vi "Set Busy Cursor.vi"() -> ()   [LabVIEW 2023]
doc: "This VI demonstrates how to set the cursor to the busy cursor. Clicking the Set Busy button will change the cursor to the busy cursor. You will still be able to click on other buttons on the user interface. Clicking the Set Busy and Disable button will set the cursor to busy and disable the cursor. During this time, all user interface events will be ignored. After 5 seconds, Unset Busy.vi will be called and the cursor will no longer be busy.\n\nThe default and busy cursors are going to be OS dependent. If a cursor that does not depend on OS is needed, Set Cursor.vi should be used instead of Set/Unset Busy. In this case, you will not be able to disable clicking.\n\nIn a real application, if the cursor is set to disable clicking, there should be some way to ensure that Unset Busy.vi can be called. Otherwise, the only way to stop the VI is to use the Abort Execution button. \n\nThis example shows a usage of the Simple State Machine project template."
uses:
  controls/Set Busy Cursor State.ctl
panel:
  out "Busy Progress":u32(slide) scale=0.0..5000.0
  in  "Button":bool
  in  "Set Busy and Disable":bool
  in  "Stop":bool
  in  "Set Busy":bool
  # "Overview: Demonstrates the use of the Cursor VIs to set a busy cursor.\nInstructions:\n1. Run the VI.\n2. Click the Set Busy button. While the Busy Progress bar is incrementing, click the Button. Notice that its value changes.\n3. After the Busy Progress is complete, click the Set Busy and Disable button. While the Busy Progress bar is incrementing, click the Button. Since busy cursor clicks are disabled, the value will not change.\n4. Click Stop to stop the VI."
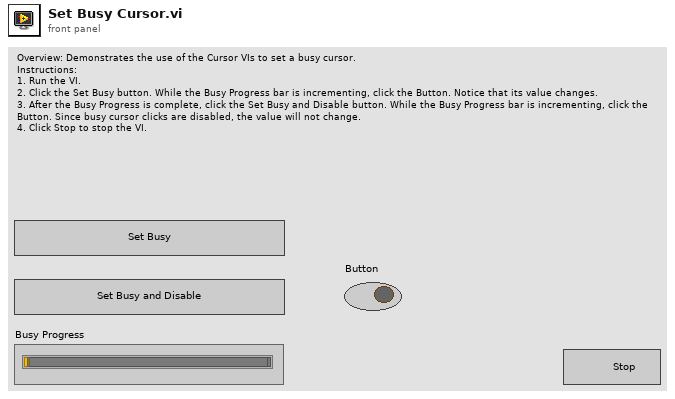
[diagram p1: front panel]
types:
  T1 = typedef "Set Busy Cursor State.ctl" = enum16{"Initialize", "Wait for Event", "Monitor Button", "Exit"}
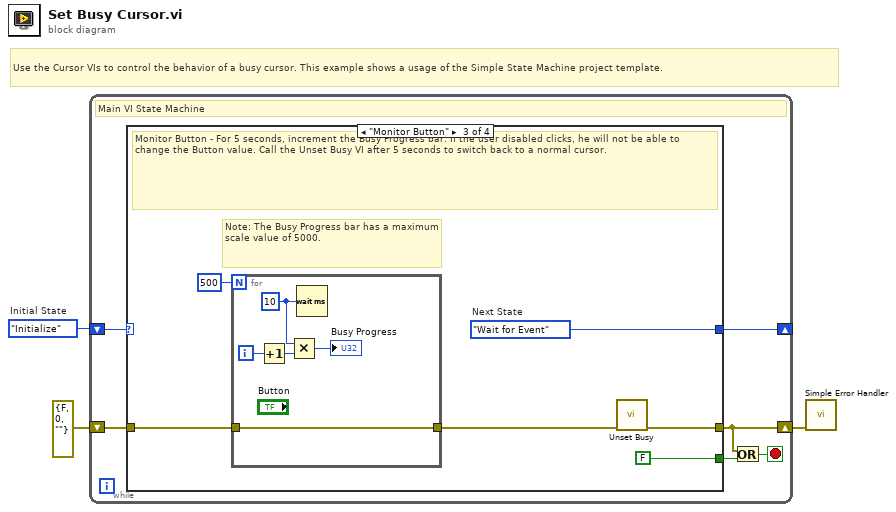
[diagram p0: block diagram]
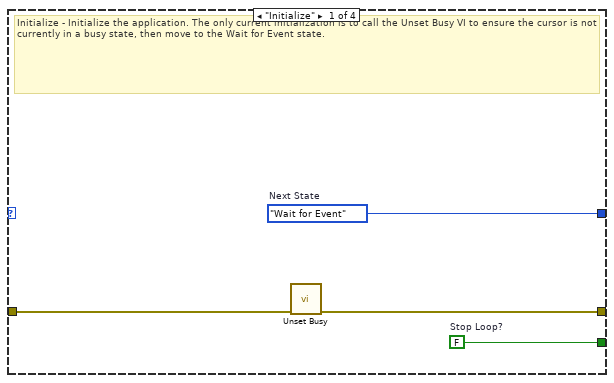
[diagram p2: hidden frame]
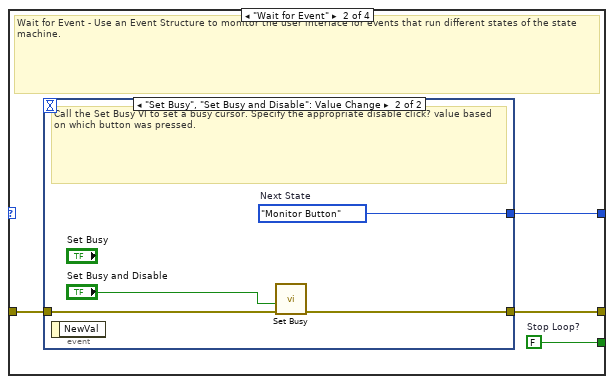
[diagram p3: hidden frame]
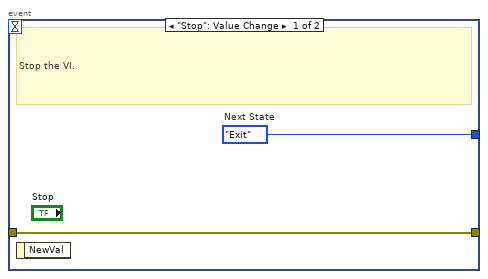
[diagram p4: hidden frame]
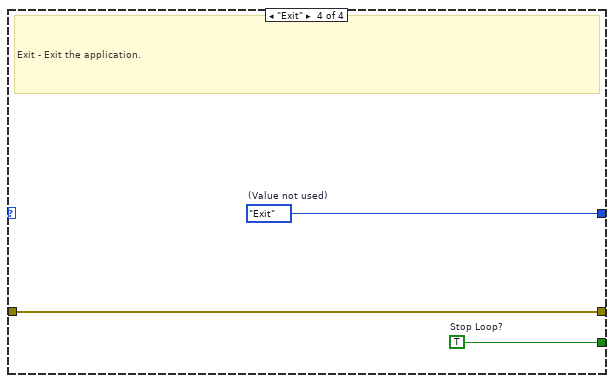
[diagram p5: hidden frame]
diagram:
  w3 = Set_Busy_Cursor_State."Initialize"  # Initial State
  # "Use the Cursor VIs to control the behavior of a busy cursor. This example shows a usage of the Simple State Machine project template."
  n1 = while {
    shift-right: [w8] -> _
    shift-left: w3 -> [w9]
    shift-right: [w4] -> w1
    shift-left: errorcluster {"status"=FALSE, "code"=0, "source"=""} ("error constant") -> [w7]
    stop <- w5 stop-if-true
    # "Main VI State Machine"
    n2 = case shown="\"Monitor Button\"" w9 {
      tunnel: [w10 w17 w24 w35] -> w8
      tunnel: [w13 w16 FALSE ("Stop Loop?") w37] -> w6
      tunnel: w7 -> [w12 w15 w27 w36]
      tunnel: [w11 w14 w28 w36] -> w4
      frame "Initialize" {
        w10 = Set_Busy_Cursor_State."Wait for Event"  # Next State
        w13 = FALSE  # Stop Loop?
        # "Initialize - Initialize the application. The only current initialization is to call the Unset Busy VI to ensure the cursor is not currently in a busy state, then move to the Wait for Event state."
        n3 = call <vilib>:"Unset Busy.vi"("error in (no error)"=w12) -> ("error out"=w11:errorcluster)  [unwired: 10 in]
      }
      frame "Wait for Event" {
        w16 = FALSE  # Stop Loop?
        # "Wait for Event - Use an Event Structure to monitor the user interface for events that run different states of the state machine."
        n4 = event shown="[1] \"Set Busy\", \"Set Busy and Disable\": Value Change" {
          selector: _ -> [_ _]
          dyn-events: _ -> [_ _]
          timeout: _ -> [_ _]
          tunnel: [w18 w20] -> w17
          tunnel: w15 -> [w19 w23]
          tunnel: [w19 w22] -> w14
          event "Stop": Value Change {
            w18 = Set_Busy_Cursor_State."Exit"  # Next State
            # "Stop the VI."
            n5 = event-data() -> ()  [unwired: 1 in, 1 out]
          }
          event "Set Busy", "Set Busy and Disable": Value Change {
            w20 = Set_Busy_Cursor_State."Monitor Button"  # Next State
            # "Call the Set Busy VI to set a busy cursor. Specify the appropriate disable click? value based on which button was pressed."
            n6 = event-data() -> ()  [unwired: 1 in, 1 out]
            n7 = call <vilib>:"Set Busy.vi"("error in (no error)"=w23, "disable click? (T)"="Set Busy and Disable") -> ("error out"=w22:errorcluster)  [unwired: 8 in, 1 out]
          }
        }
      }
      frame "Monitor Button" {
        w24 = Set_Busy_Cursor_State."Wait for Event"  # Next State
        # "Note: The Busy Progress bar has a maximum scale value of 5000."
        # "Monitor Button - For 5 seconds, increment the Busy Progress bar. If the user disabled clicks, he will not be able to change the Button value. Call the Unset Busy VI after 5 seconds to switch back to a normal cursor."
        n8 = for {
          N: 500 -> [_]
          tunnel: w27 -> [w30]
          tunnel: [w30] -> w25
          i -> [w34]
          w32 = u32 10 ("milliseconds to wait")
          n9 = Increment(x=w34) -> (x+1=w33:i32)
          n10 = Multiply(x=w32, y=w33) -> (x*y=→"Busy Progress":u32)
          n11 = Wait (ms)(milliseconds to wait=w32) -> ()  [unwired: 1 out]
        }
        n12 = call <vilib>:"Unset Busy.vi"("error in (no error)"=w25) -> ("error out"=w28:errorcluster)  [unwired: 10 in]
      }
      frame "Exit" {
        w35 = Set_Busy_Cursor_State."Exit"  # (Value not used)
        w37 = TRUE  # Stop Loop?
        # "Exit - Exit the application."
      }
    }
    n13 = Or(x=w4, y=w6) -> (x .or. y?=w5:bool)
  }
  n14 = call <vilib>:"Simple Error Handler.vi"("error in (no error)"=w1) -> ()  [unwired: 4 in, 5 out]
